vi "Create.vi"(8 "error in (no error)":errorcluster, 10 "Debugger":refnum<class "Debugger.lvclass">, 11 "Messages Composite View In":refnum<class "Messages Composite View.lvclass">) -> (0 "error out":errorcluster, 3 "Messages Composite View Out":refnum<class "Messages Composite View.lvclass">)   [LabVIEW 2020, in "Messages Composite View.lvclass"]
uses:
  Messages Composite View.lvclass
  Debugger/Debugger.lvclass
  C:/Users/anton/Documents/GitHub/triarc-debugger/source/Process/Debug Process.lvclass
  List Seen Messages View Model/List Messages View Model.lvclass
  C:/Users/anton/Documents/GitHub/triarc-debugger/source/List Box View Model_/List Box View Model.lvclass
  List View/Messages List Box View.lvclass
  C:/Users/anton/Documents/GitHub/triarc-debugger/source/Debug View/Debug View.lvclass
  Multicolumn List Box View/Multicolumn List Box View.lvclass
  Multicolumn List Box View Model/Multicolumn List Box View Model.lvclass
  Variant View/Variant View.lvclass
  Variant View Model/Variant View Model.lvclass
  Control View/Control View.lvclass
  Debug View/Debug View.lvclass/Debug View.ctl
  Variant View/Variant View.lvclass/Variant View.ctl
  Multicolumn List Box View/Multicolumn List Box View.lvclass/Multicolumn List Box View.ctl
  List View/Messages List Box View.lvclass/Messages List Box View.ctl
  Messages Composite View.lvclass/Messages Composite View.ctl
  List Seen Processes View Model/List Processes View Model.lvclass
  Debug View/Debug View.lvclass
  C:/Users/anton/Documents/GitHub/triarc-debugger/source/Variant View/Variant View.lvclass
  C:/Users/anton/Documents/GitHub/triarc-debugger/source/Control View/Control View.lvclass
  C:/Users/anton/Documents/GitHub/triarc-debugger/source/Multicolumn List Box View/Multicolumn List Box View.lvclass
  Process List Box View/Processes List Box View.lvclass
  C:/Users/anton/Documents/GitHub/triarc-debugger/source/List Seen Messages View Model/List Messages View Model.lvclass
  C:/Users/anton/Documents/GitHub/triarc-debugger/source/Debugger/Debugger.lvclass
  C:/Users/anton/Documents/GitHub/triarc-debugger/source/Debug Data Event/Debug Data Listener.lvclass
  C:/Users/anton/Documents/GitHub/triarc-debugger/source/List Seen Processes View Model/List Processes View Model.lvclass
  C:/Users/anton/Documents/GitHub/triarc-debugger/source/Process List Box View/Processes List Box View.lvclass
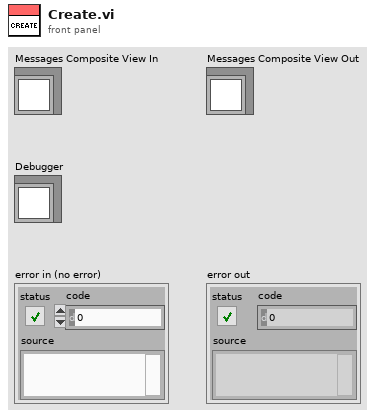
[diagram p1: front panel]
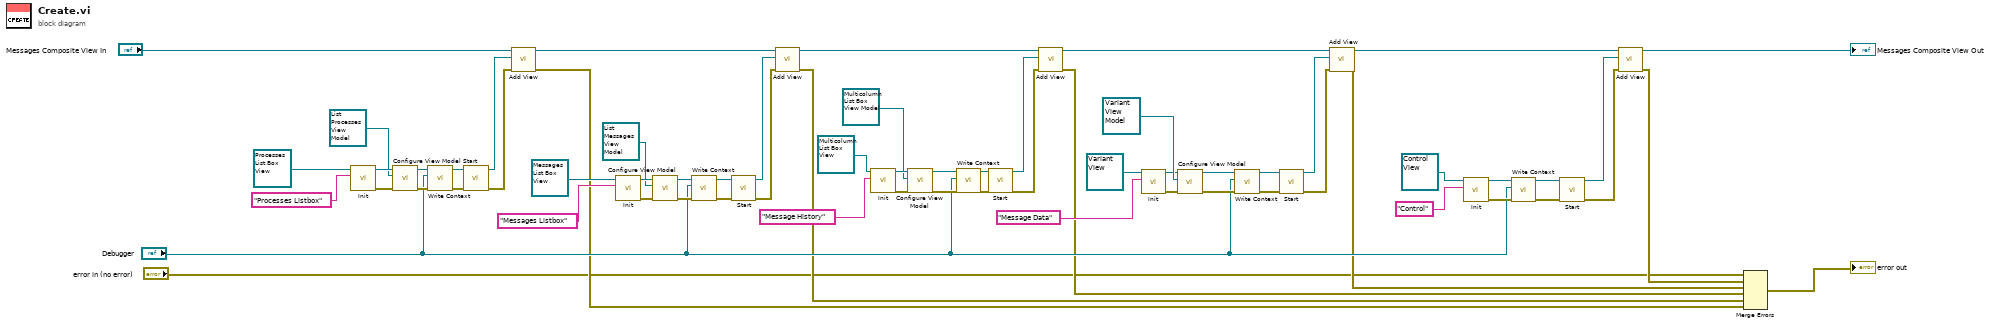
[diagram p0: block diagram]
diagram:
  n1 = call-dynamic "Init.vi"("Name"="Processes Listbox", "Debug View In"=refnum<class "Processes List Box View.lvclass"> refnum ("Processes List Box View.lvclass")) -> ("error out"=w54:errorcluster, "Debug View Out"=w55:refnum<class "Processes List Box View.lvclass">)  [unwired: 8 in]
  n2 = call "Configure View Model.vi"("error in (no error)"=w54, "List Box View Model"=refnum<class "List Processes View Model.lvclass"> refnum ("List Processes View Model.lvclass"), "List Box View In"=w55) -> ("error out"=w53:errorcluster, "List Box View Out"=w22:refnum<class "Processes List Box View.lvclass">)  [unwired: 7 in]
  n3 = call "Write Context.vi"("error in (no error)"=w53, "Debug Process.lvclass"="Debugger", "Debug View In"=w22) -> ("error out"=w23:errorcluster, "Debug View Out"=w21:refnum<class "Processes List Box View.lvclass">)  [unwired: 7 in]
  n4 = call "Start.vi"("error in (no error)"=w23, "Debug View In"=w21) -> ("error out"=w58:errorcluster, "Debug View In"=w59:refnum<class "Processes List Box View.lvclass">)  [unwired: 8 in]
  n5 = call "Add View.vi"("error in (no error)"=w58, "Debug Process"=w59, "Messages Composite View In"="Messages Composite View In") -> ("error out"=w3:errorcluster, "Messages Composite View In"=w61:refnum<class "Messages Composite View.lvclass">)  [unwired: 7 in]
  n6 = call-dynamic "Init.vi"("Name"="Messages Listbox", "Debug View In"=refnum<class "Messages List Box View.lvclass"> refnum ("List Box View.lvclass")) -> ("error out"=w64:errorcluster, "Debug View Out"=w50:refnum<class "Messages List Box View.lvclass">)  [unwired: 8 in]
  n7 = call "Configure View Model.vi"("error in (no error)"=w64, "List Box View Model"=refnum<class "List Messages View Model.lvclass"> refnum ("List Messages View Model.lvclass"), "List Box View In"=w50) -> ("error out"=w51:errorcluster, "List Box View Out"=w19:refnum<class "Messages List Box View.lvclass">)  [unwired: 7 in]
  n8 = call "Write Context.vi"("error in (no error)"=w51, "Debug Process.lvclass"="Debugger", "Debug View In"=w19) -> ("error out"=w20:errorcluster, "Debug View Out"=w18:refnum<class "Messages List Box View.lvclass">)  [unwired: 7 in]
  n9 = call "Start.vi"("error in (no error)"=w20, "Debug View In"=w18) -> ("error out"=w57:errorcluster, "Debug View Out"=w56:refnum<class "Messages List Box View.lvclass">)  [unwired: 8 in]
  n10 = call "Add View.vi"("error in (no error)"=w57, "Debug Process"=w56, "Messages Composite View In"=w61) -> ("error out"=w4:errorcluster, "Messages Composite View Out"=w60:refnum<class "Messages Composite View.lvclass">)  [unwired: 7 in]
  n11 = call-dynamic "Init.vi"("Name"="Message History", "Debug View In"=refnum<class "Multicolumn List Box View.lvclass"> refnum ("Multicolumn List Box View In")) -> ("error out"=w48:errorcluster, "Debug View Out"=w45:refnum<class "Multicolumn List Box View.lvclass">)  [unwired: 8 in]
  n12 = call "Configure View Model.vi"("error in (no error)"=w48, "View Model"=refnum<class "Multicolumn List Box View Model.lvclass"> refnum ("Multicolumn List Box View Model.lvclass"), "Multicolumn List Box View In"=w45) -> ("error out"=w47:errorcluster, "Multicolumn List Box View Out"=w16:refnum<class "Multicolumn List Box View.lvclass">)  [unwired: 7 in]
  n13 = call "Write Context.vi"("error in (no error)"=w47, "Debug Process.lvclass"="Debugger", "Debug View In"=w16) -> ("error out"=w17:errorcluster, "Debug View Out"=w15:refnum<class "Multicolumn List Box View.lvclass">)  [unwired: 7 in]
  n14 = call "Start.vi"("error in (no error)"=w17, "Debug View In"=w15) -> ("error out"=w42:errorcluster, "Debug View Out"=w43:refnum<class "Multicolumn List Box View.lvclass">)  [unwired: 8 in]
  n15 = call "Add View.vi"("error in (no error)"=w42, "Debug Process"=w43, "Messages Composite View In"=w60) -> ("error out"=w5:errorcluster, "Messages Composite View Out"=w32:refnum<class "Messages Composite View.lvclass">)  [unwired: 7 in]
  n16 = call-dynamic "Init.vi"("Name"="Message Data", "Debug View In"=refnum<class "Variant View.lvclass"> refnum ("Multicolumn List Box View In")) -> ("error out"=w33:errorcluster, "Debug View Out"=w36:refnum<class "Variant View.lvclass">)  [unwired: 8 in]
  n17 = call "Configure View Model.vi"("error in (no error)"=w33, "List Box View Model"=refnum<class "Variant View Model.lvclass"> refnum ("Variant View Model.lvclass"), "List Box View In"=w36) -> ("error out"=w34:errorcluster, "List Box View Out"=w13:refnum<class "Variant View.lvclass">)  [unwired: 7 in]
  n18 = call "Write Context.vi"("error in (no error)"=w34, "Debug Process.lvclass"="Debugger", "Debug View In"=w13) -> ("error out"=w14:errorcluster, "Debug View Out"=w12:refnum<class "Variant View.lvclass">)  [unwired: 7 in]
  n19 = call "Start.vi"("error in (no error)"=w14, "Debug View In"=w12) -> ("error out"=w39:errorcluster, "Debug View Out"=w38:refnum<class "Variant View.lvclass">)  [unwired: 8 in]
  n20 = call "Add View.vi"("error in (no error)"=w39, "Debug Process"=w38, "Messages Composite View In"=w32) -> ("error out"=w6:errorcluster, "Messages Composite View Out"=w27:refnum<class "Messages Composite View.lvclass">)  [unwired: 7 in]
  n21 = call-dynamic "Init.vi"("Name"="Control", "Debug View In"=refnum<class "Control View.lvclass"> refnum ("Control View.lvclass")) -> ("error out"=w31:errorcluster, "Debug View Out"=w10:refnum<class "Control View.lvclass">)  [unwired: 8 in]
  n22 = call "Write Context.vi"("error in (no error)"=w31, "Debug Process.lvclass"="Debugger", "Debug View In"=w10) -> ("error out"=w11:errorcluster, "Debug View Out"=w9:refnum<class "Control View.lvclass">)  [unwired: 7 in]
  n23 = call "Start.vi"("error in (no error)"=w11, "Debug View In"=w9) -> ("error out"=w29:errorcluster, "Debug View Out"=w30:refnum<class "Control View.lvclass">)  [unwired: 8 in]
  n24 = call "Add View.vi"("error in (no error)"=w29, "Debug Process"=w30, "Messages Composite View In"=w27) -> ("error out"=w25:errorcluster, "Messages Composite View Out"=→"Messages Composite View Out":refnum<class "Messages Composite View.lvclass">)  [unwired: 7 in]
  n25 = Merge Errors("error in (no error)", w25, w6, w5, w4, w3) -> (→"error out":errorcluster)
